vi "Read Counter Driven State.vi"(8 "error in":errorcluster, 11 "counter driven output channel in":refnum<class "Counter Driven Output Channel.lvclass">) -> (0 "error out":errorcluster, 2 "counter driven state":T1, 3 "counter driven output channel out":refnum<class "Counter Driven Output Channel.lvclass">)   [LabVIEW 2020, in "Scan Engine Scripting.lvlib" / "Counter Driven Output Channel.lvclass"]
uses:
  Counter Driven Output Channel.lvclass
  Counter Driven State.ctl
  Counter Driven Output Channel.lvclass/Counter Driven Output Channel.ctl
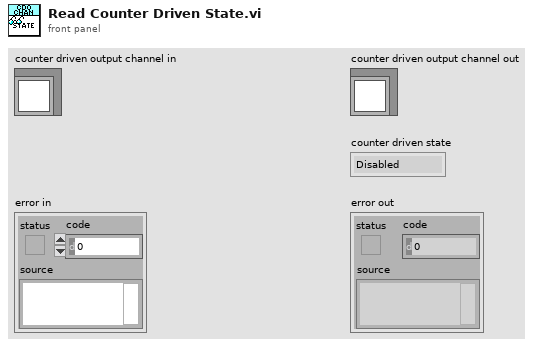
[diagram p1: front panel]
types:
  T1 = typedef "Scan Engine Scripting.lvlib/Counter Driven Output Channel.lvclass/Counter Driven State.ctl" = enum16{"Disabled", "Enabled"}
  T2 = typedef "Scan Engine Scripting.lvlib/Copy of Counter Driven Output Channel.lvclass/Counter Driven State.ctl" = enum16{"Disabled", "Enabled"}
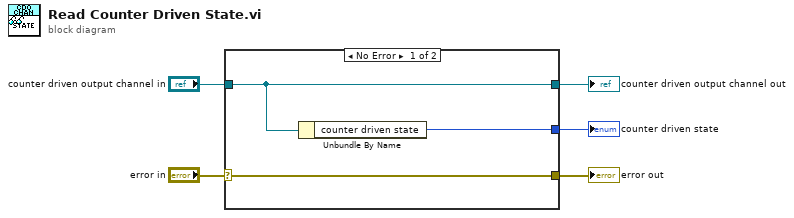
[diagram p0: block diagram]
diagram:
  n1 = case shown="No Error" "error in" {
    selector: "error in" -> [w8 w9]
    tunnel: [w8 w9] -> w4
    tunnel: [w7 w10] -> w2
    tunnel: "counter driven output channel in" -> [w7 w10]
    tunnel: [w6 _] -> w1
    frame No Error {
      n2 = Unbundle By Name(w7) -> ("counter driven state"=w6:T2)
    }
    frame Error {
    }
  }
  "error out" <- w4
  "counter driven output channel out" <- w2
  "counter driven state" <- w1
